vi "Data-ConvertSPCtoPhotInfo.vi"() -> ()   [LabVIEW 2023]
doc: "This VI demonstrates how a *.spc file filled with raw event data from a SPC_read_fifo call can be converted to a PhotInfo-cluster (structure) and written to a file in the Becker&Hickl propriety format *.ph. \n\ninfo@becker-hickl.com"
uses:
  SPC_Wrappers/SPC_Controls/SPC_PhotInfo.ctl
  SPC_Wrappers/SPC_Controls/WhatToRead.ctl
  SPC_Wrappers/SPC_Controls/ModuleTypes.ctl
  SPC_Wrappers/SPC_Controls/Fifo_Type.ctl
panel:
  out "EventHeader":u32 format="%08x"
  out "Macro Time Clk":dbl caption="ns"
  in  "SPC-FilePath":path
  out "PhotInfo32":T1[](array[typedef]) {"Flags" max=3 format="%016b"; "Routing channel" step=1; "Micro time value" step=1; "Macro time clocks high" step=1; "Macro time clocks low" step=1}
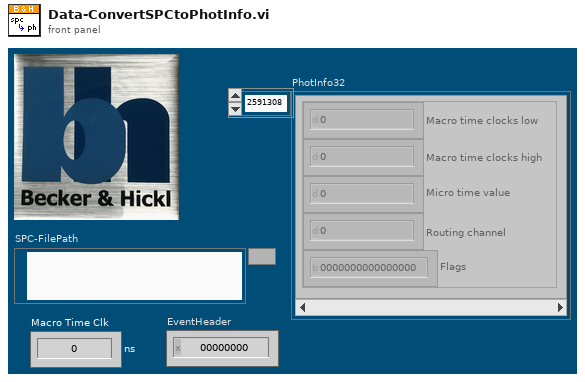
[diagram p1: front panel]
types:
  T1 = typedef "SPC_PhotInfo.ctl" = cluster{"Macro time clocks low":u32, "Macro time clocks high":u32, "Micro time value":u16, "Routing channel":u16, "Flags":u16}
  T2 = enum16{"big-endian, network order", "native, host order", "little-endian"}
  T3 = enum16{"open", "replace", "create", "open or create", "replace or create", "replace or create with confirmation"}
  T4 = typedef "Fifo_Type.ctl" = i16
  T5 = typedef "ModuleTypes.ctl" = i16
  T6 = typedef "WhatToRead.ctl" = cluster{"Valid Photons":bool, "Invalid Photons":bool, "Pixel":bool, "Line":bool, "Frame":bool, "Marker 3":bool}
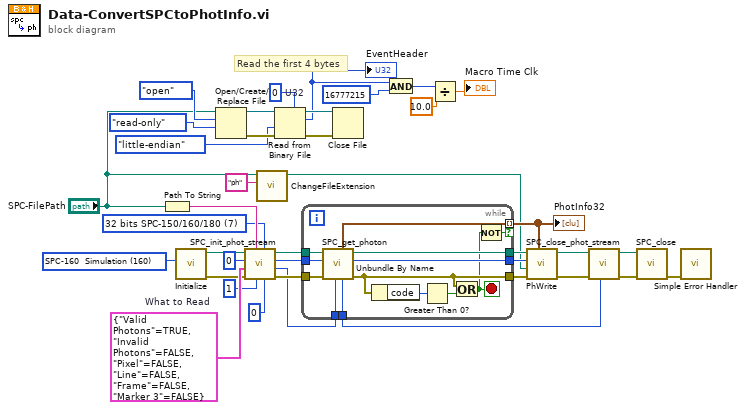
[diagram p0: block diagram]
diagram:
  w10 = u32 0  # U32
  w15 = T4 7 items=["48 bits SPC-6x0"=2, "32 bits SPC-6x0"=3, "32 bits SPC-130"=4, "32 bits SPC-830"=5, "32 bits SPC-140"=6, "32 bits SPC-150/160/180"=7, "32 bits DPC-230"=8, "32 bits FIFO_IMAGE"=9, "FIFO_D590"=10, "FIFO_TDC"=11, "FIFO_TDC_ABS"=12] ("fifo_type")
  w16 = T5 160 items=["Hardware Modus"=0, "SPC-600 Simulation"=600, "SPC-630 Simulation"=630, "SPC-700  Simulation"=700, "SPC-730  Simulation"=730, "SPC-130  Simulation"=130, "SPC-830  Simulation"=830, "SPC-140  Simulation"=140, "SPC-930  Simulation"=930, "DPC-230  Simulation"=230, "SPC-150  Simulation"=150, "SPC-150 N  Simulation"=151, "SPC-150 NX  Simulation"=152, "SPC-130 EM  Simulation"=131, "SPC-130 EMN  Simulation"=132, "SPC-160  Simulation"=160, "SPC-160 X  Simulation"=161, "SPC-160 PCIE  Simulation"=162, "DPC-330  Simulation"=330, "DPC 590  Simulation"=590] ("Modul Type to Simulate")
  w37 = T6 {"Valid Photons"=TRUE, "Invalid Photons"=FALSE, "Pixel"=FALSE, "Line"=FALSE, "Frame"=FALSE, "Marker 3"=FALSE}  # What to Read
  # "Read the first 4 bytes"
  n1 = Path To String(path="SPC-FilePath") -> (string=w39:string)
  n2 = call "Initialize.vi"("Modul Type to Simulate"=w16) -> ("ErrorOut"=w28:errorcluster, "DLL Path"=w29:path)  [unwired: 6 in, 3 out]
  n3 = Open/Create/Replace File(file path (use dialog)="SPC-FilePath", operation (0:open)=T3."open", access (0:read/write)=enum16{"read/write", "read-only", "write-only"}."read-only") -> (refnum out=w9:refnum<file>, error out=w8:errorcluster)  [unwired: 3 in, 1 out]
  n4 = call "SPC_init_phot_stream.vi"("#files_to_use"=i16 0, "fifo_type"=w15, "stream_type"=i16 1, "spc_file"=w39, "Error In"=w28, "what_to_read"=w37, "Modul No"=i16 0, "DLL Path"=w29) -> ("Error Out"=w32:errorcluster, "Stream Handle"=w31:i16, "Modul No"=w34:i16, "DLL Path"=w33:path)
  n5 = call "ChangeFileExtension.vi"("NewExtension"="ph", "OldPath"="SPC-FilePath") -> ("NewPath"=w18:path)  [unwired: 8 in, 1 out]
  n6 = Read from Binary File(5:w10, 8:w8, 9:T2."little-endian" ("byte order (0:big-endian, network order)"), 11:w9) -> (0:w4:errorcluster, 2:w2:u32, 3:w3:refnum<file>)  [unwired: 2 in, 1 out]
  "EventHeader" <- w2
  n7 = while {
    tunnel: w34 -> [w52]
    tunnel: w31 -> [w49]
    tunnel: [w47] -> w30
    tunnel: w33 -> [w51]
    tunnel: [w48] -> w23
    tunnel: w32 -> [w50]
    tunnel: [w43] -> w25
    tunnel: [w46] -> w21 mode=indexing if=w40
    tunnel: [w42] -> w24
    stop <- w41 stop-if-true
    n8 = call "SPC_get_photon.vi"("Stream Handle"=w49, "Error In"=w50, "Module No"=w52, "DLL Path"=w51) -> ("Error Out"=w43:errorcluster, "Module No"=w42:i16, "DLL Path"=w48:path, "Stream Handle"=w47:i16, "PhotInfo"=w46:T1)  [unwired: 3 in]
    n9 = Unbundle By Name(w43) -> ("code"=w45:i32)
    n10 = Greater Than 0?(x=w45) -> (x > 0?=w44:bool)
    n11 = Or(x=w43, y=w44) -> (x .or. y?=w41:bool)
    n12 = Not(x=w41) -> (.not. x?=w40:bool)
  }
  "PhotInfo32" <- w21
  n13 = Close File(refnum=w3, error in=w4) -> ()  [unwired: 2 out]
  n14 = And(x=w2, y=u32 16777215) -> (x .and. y?=w12:u32)
  n15 = Divide(x=w12, y=10.0) -> (x/y=→"Macro Time Clk":dbl)
  n16 = call "PhWrite.vi"("PhotInfo32"=w21, "Error In"=w25, "PhFilePath"=w18, "Module No"=w24, "DLL Path"=w23) -> ("error out"=w22:errorcluster, "DLL Path"=w20:path)  [unwired: 5 in]
  n17 = call "SPC_close_phot_stream.vi"("Stream Handle"=w30, "Error In"=w22, "DLL Path"=w20) -> ("Error Out"=w26:errorcluster, "DLL Path"=w27:path)  [unwired: 6 in, 1 out]
  n18 = call "SPC_close.vi"("Error In"=w26, "DLL Path"=w27) -> ("Error Out"=w17:errorcluster)  [unwired: 8 in, 1 out]
  n19 = call <vilib>:"Simple Error Handler.vi"("error in (no error)"=w17) -> ()  [unwired: 4 in, 5 out]
